vi "布尔控件讲解.vi"() -> ()   [LabVIEW 2018]
panel:
  out "结果":bool
  in  "复合运算 3":bool
  in  "复合运算 2":bool
  in  "复合运算":bool
  out "x与y？":bool
  in  "与运算 2":bool
  in  "与运算":bool
  out "显示开关":bool
  in  "控制LED":bool
  out "电源指示灯":bool
  out "布尔 2":bool
  in  "布尔":bool
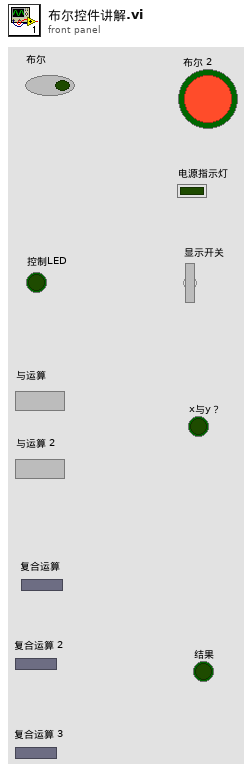
[diagram p1: front panel]
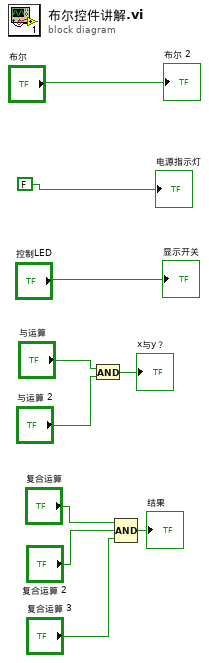
[diagram p0: block diagram]
diagram:
  n1 = And(x="与运算", y="与运算 2") -> (x .and. y?=→"x与y？":bool)
  n2 = Compound Arithmetic op=AND ("复合运算")("复合运算", "复合运算 2", "复合运算 3") -> (→"结果":bool)
  "布尔 2" <- "布尔"
  "电源指示灯" <- FALSE
  "显示开关" <- "控制LED"
